vi "Exemplos.vi"() -> ()   [LabVIEW 2014]
uses:
  <vilib>/Utility/file.llb/Write To Spreadsheet File (DBL).vi
  <vilib>/Utility/file.llb/Read From Spreadsheet File (string).vi
  <vilib>/gmath/NI_Gmath.lvlib
panel:
  out "number":dbl[][](array[numeric])
  out "all rows":string[][](array[string])
  out "xi used":dbl[](array[numeric]) format="%_6g"
  out "yi":dbl[](array[numeric]) format="%_6g"
  out "XY Graph":cluster{"xi used":dbl[], "yi":dbl[]}[](graph)
  out "Array 2":dbl[](array[numeric])
  out "Array":i32[](array[numeric])
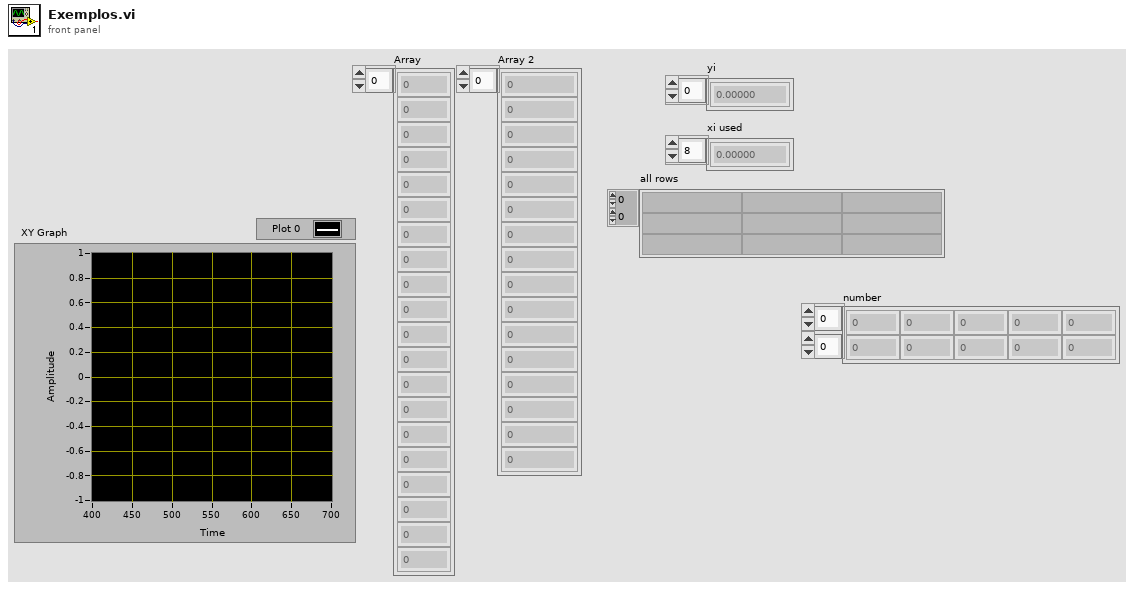
[diagram p1: front panel]
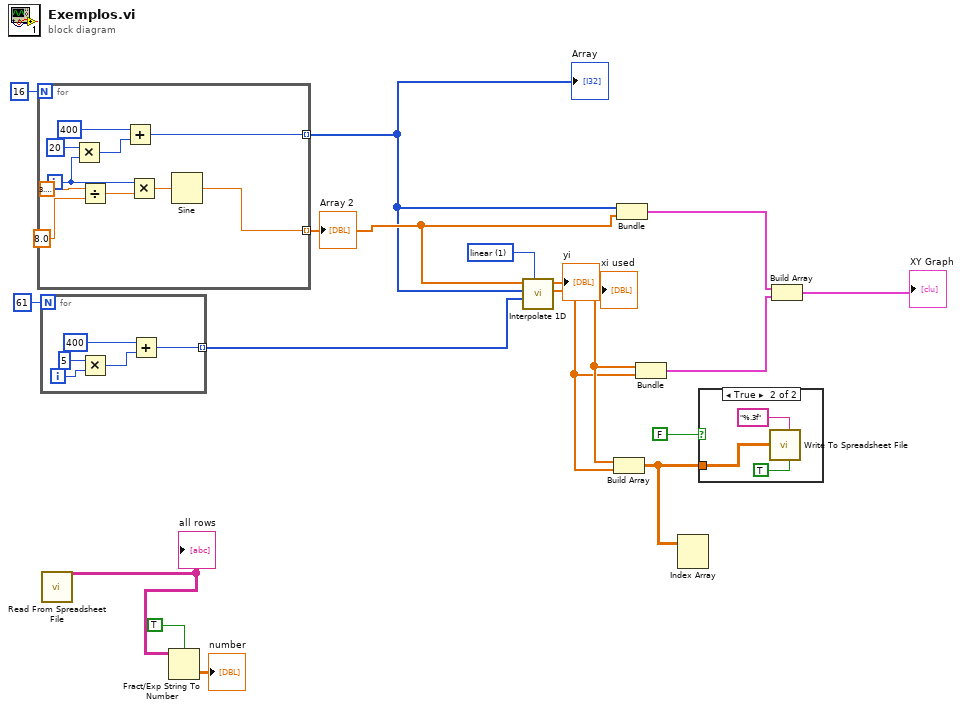
[diagram p0: block diagram]
diagram:
  w13 = 1 items=["nearest", "linear", "spline", "cubic Hermite", "Lagrange"] ("method")
  n1 = for {
    N: 16 -> [_]
    tunnel: [w23] -> w14 mode=indexing
    tunnel: [w17] -> w15 mode=indexing
    i -> [w22]
    n2 = Multiply(x=20, y=w22) -> (x*y=w24:i32)
    n3 = Divide(x=3.141592653589793, y=8.0) -> (x/y=w19:dbl)
    n4 = Add(x=400, y=w24) -> (x+y=w23:i32)
    n5 = Multiply(x=w22, y=w19) -> (x*y=w18:dbl)
    n6 = Sine(x=w18) -> (sin(x)=w17:dbl)
  }
  "Array" <- w14
  "Array 2" <- w15
  n7 = for {
    N: 61 -> [_]
    tunnel: [w27] -> w11 mode=indexing
    i -> [w28]
    n8 = Multiply(x=5, y=w28) -> (x*y=w29:i32)
    n9 = Add(x=400, y=w29) -> (x+y=w27:i32)
  }
  n10 = call-poly <vilib>:"Read From Spreadsheet File.vi"() -> ("all rows"=w4:string[][])  [unwired: 7 in, 4 out]
  "all rows" <- w4
  n11 = Fract/Exp String To Number(use system decimal point (T)=TRUE, string=w4) -> (number=→"number":dbl[][])  [unwired: 2 in, 1 out]
  n12 = call <vilib>:"Interpolate 1D.vi"("method"=w13, "xi"=w11, "X"=w14, "Y"=w15) -> ("xi used"=w7:dbl[], "yi"=w6:dbl[])  [unwired: 5 in, 1 out]
  "yi" <- w6
  "xi used" <- w7
  n13 = Build Array(w7, w6) -> (w5:dbl[][])
  n14 = Bundle(w14, w15) -> (w1:cluster{i32[], dbl[]})  [unwired: 1 in]
  n15 = Bundle("xi used"=w7, "yi"=w6) -> (w10:cluster{"xi used":dbl[], "yi":dbl[]})  [unwired: 1 in]
  n16 = Index Array(array=w5) -> ()  [unwired: 2 in, 1 out]
  n17 = case shown="True" FALSE {
    tunnel: w5 -> [_ w32]
    frame False {
    }
    frame True {
      n18 = call-poly <vilib>:"Write To Spreadsheet File.vi"("transpose? (no:F)"=TRUE, "format (%.3f)"="%.3f", "2D data"=w32) -> ()  [unwired: 5 in, 1 out]
    }
  }
  n19 = Build Array(w1, w10) -> (→"XY Graph":cluster{"xi used":dbl[], "yi":dbl[]}[])
